vi "RFController getDPDKKPI.vi"(6 "contextId":T1, 8 "error in":errorcluster, 9 "timeout (ms)":i32=-1, 10 "Request Data":T4, 11 "gRPC ID":T1) -> (0 "error out":errorcluster, 2 "Response Data":T2, 3 "gRPC ID out":T1)   [LabVIEW 2024, in "FlexCompute_grpc_client.lvlib"]
uses:
  FlexCompute_grpc_client.lvlib
  <vilib>/gRPC/LabVIEW gRPC Library/Shared/grpcId.ctl
  RPC Messages/rfcontrol_Empty.ctl
  RPC Messages/rfcontrol_KPIData.ctl
  RPC Messages/rfcontrol_Status.ctl
  RPC Messages/rfcontrol_KPIData_Flat.ctl
  14035477-4c25-4107-8ed5-d0c4ef420ce5.vi
  <vilib>/gRPC/LabVIEW gRPC Library/Shared/TranslateGrpcError.vi
  <vilib>/gRPC/LabVIEW gRPC Library/Shared/Wait On Occurrence.vi
  <vilib>/gRPC/LabVIEW gRPC Library/Shared/Is Feature Enabled.vi
  <vilib>/gRPC/LabVIEW gRPC Library/Server API/Server/Get Server DLL Path.vi
  <vilib>/Utility/error.llb/Error Cluster From Error Code.vi
  <vilib>/gRPC/LabVIEW gRPC Library/grpc-lvsupport-release.lvlib
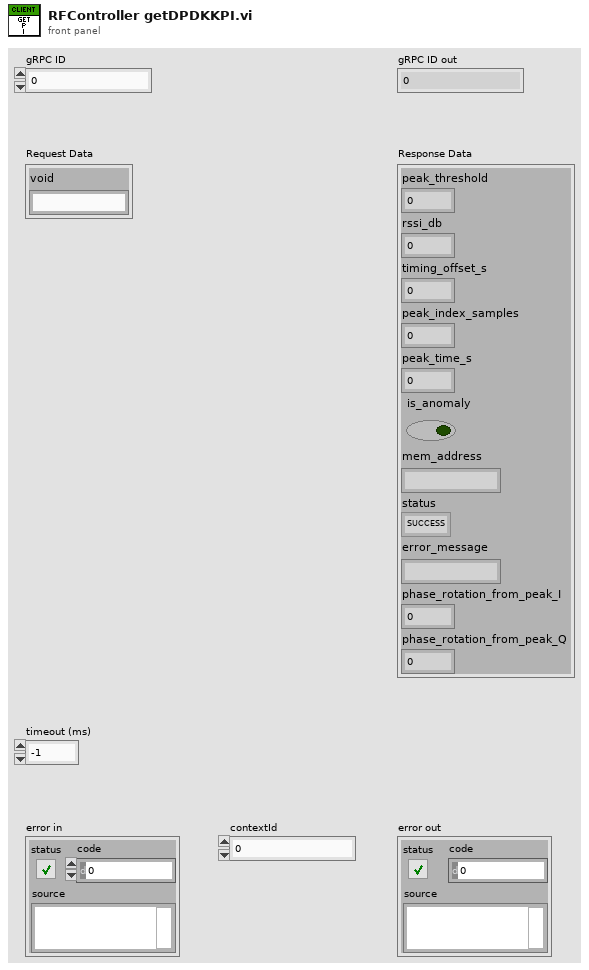
[diagram p1: front panel]
types:
  T1 = typedef "grpc-lvsupport-release.lvlib/grpcId.ctl" = u64
  T2 = typedef "FlexCompute_grpc_client.lvlib/rfcontrol_KPIData.ctl" = cluster{"peak_threshold":dbl, "rssi_db":dbl, "timing_offset_s":dbl, "peak_index_samples":i32, "peak_time_s":dbl, "is_anomaly":bool, "mem_address":string, "status":T3, "error_message":string, "phase_rotation_from_peak_I":sgl, "phase_rotation_from_peak_Q":sgl}
  T3 = typedef "FlexCompute_grpc_client.lvlib/rfcontrol_Status.ctl" = enum32{"SUCCESS", "ERROR"}
  T4 = typedef "FlexCompute_grpc_client.lvlib/rfcontrol_Empty.ctl" = cluster{"void":string}
  T5 = typedef "FlexCompute_grpc_client.lvlib/rfcontrol_KPIData_Flat.ctl" = cluster{"peak_threshold":dbl, "rssi_db":dbl, "timing_offset_s":dbl, "peak_index_samples":i32, "peak_time_s":dbl, "is_anomaly":bool, "mem_address":string, "status":T3, "error_message":string, "phase_rotation_from_peak_I":sgl, "phase_rotation_from_peak_Q":sgl}
  T6 = typedef "FlexCompute_grpc_client.lvlib/rfcontrol_Empty_Flat.ctl" = cluster{"void":string}
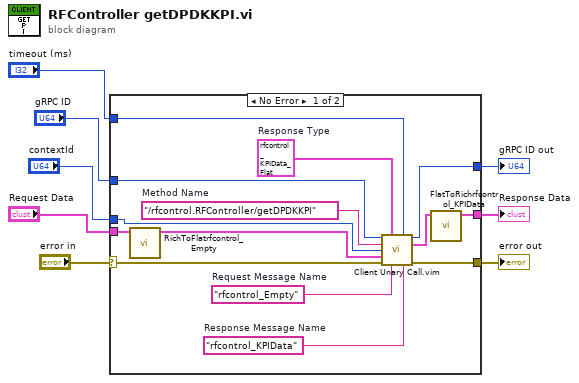
[diagram p0: block diagram]
diagram:
  n1 = case shown="No Error" "error in" {
    selector: "error in" -> [w18 w23]
    tunnel: [w17 w23] -> w7
    tunnel: "gRPC ID" -> [w16 w24]
    tunnel: [w15 w24] -> w5
    tunnel: "Request Data" -> [w12 _]
    tunnel: [w9 _] -> w3
    tunnel: "timeout (ms)" -> [w14 _]
    tunnel: "contextId" -> [w13 _]
    frame No Error {
      w19 = "rfcontrol_KPIData"  # Response Message Name
      w20 = "rfcontrol_Empty"  # Request Message Name
      w21 = T5 {"peak_threshold"=0.0, "rssi_db"=0.0, "timing_offset_s"=0.0, "peak_index_samples"=0, "peak_time_s"=0.0, "is_anomaly"=FALSE, "mem_address"="", "status"=enum."SUCCESS", "error_message"="", "phase_rotation_from_peak_I"=0.0, "phase_rotation_from_peak_Q"=0.0}  # Response Type
      w22 = "/rfcontrol.RFController/getDPDKKPI"  # Method Name
      n2 = call "RichToFlatrfcontrol_Empty.vi"("InputCluster"=w12) -> ("OutputCluster"=w11:T6)  [unwired: 10 in]
      n3 = call "Client Unary Call.vim"("ClientID in"=w16, "Response Type"=w21, "timeout (ms)"=w14, "Method Name"=w22, "contextId"=w13, "Request Data"=w11, "error in"=w18, "Request Message Name"=w20, "Response Message Name"=w19) -> ("ClientID out"=w15:u64, "Response Data"=w10:T5, "error out"=w17:errorcluster)  [unwired: 4 in]
      n4 = call "FlatToRichrfcontrol_KPIData.vi"("InputCluster"=w10) -> ("OutputCluster"=w9:T2)  [unwired: 10 in]
    }
    frame Error {
    }
  }
  "error out" <- w7
  "gRPC ID out" <- w5
  "Response Data" <- w3
